vi "Build wash Parameters.vi"(8 "error in (no error)":errorcluster, 10 "Data Controls":T2, 11 "configuration file path":path) -> (0 "error out":errorcluster, 2 "Wash Parameters Array":T1[](array[typedef]) {"Time Target" format="%0.2f"; "Car Position Slider" max=3 scale=0.0..4.0})   [LabVIEW 2015]
doc: "VI used to set parameters for each wash option chosen by the user and build and array output."
uses:
  controls/UI Data.ctl
  controls/Washing Option Parameters.ctl
  <vilib>/Utility/config.llb/Read Key (U32).vi
  <vilib>/Utility/config.llb/Read Key (Double).vi
  <vilib>/Utility/config.llb/NI_LVConfig.lvlib
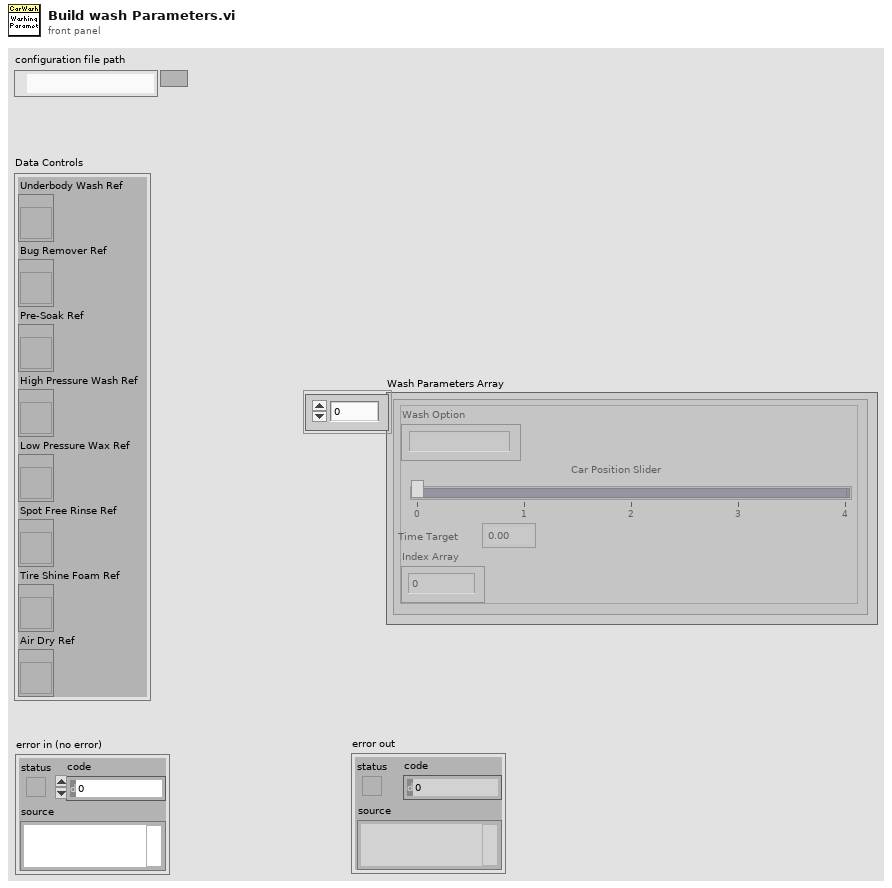
[diagram p1: front panel]
types:
  T1 = typedef "Washing Option Parameters.ctl" = cluster{"Wash Option":string, "Car Position Slider":u8, "Time Target":dbl, "Index Array":i32}
  T2 = typedef "UI Data.ctl" = cluster{"Underbody Wash Ref":refnum<vi>, "Bug Remover Ref":refnum<vi>, "Pre-Soak Ref":refnum<vi>, "High Pressure Wash Ref":refnum<vi>, "Low Pressure Wax Ref":refnum<vi>, "Spot Free Rinse Ref":refnum<vi>, "Tire Shine Foam Ref":refnum<vi>, "Air Dry Ref":refnum<vi>}
  T3 = typedef "NI_LVConfig.lvlib/Config Data RefNum.ctl" = refnum<k1>
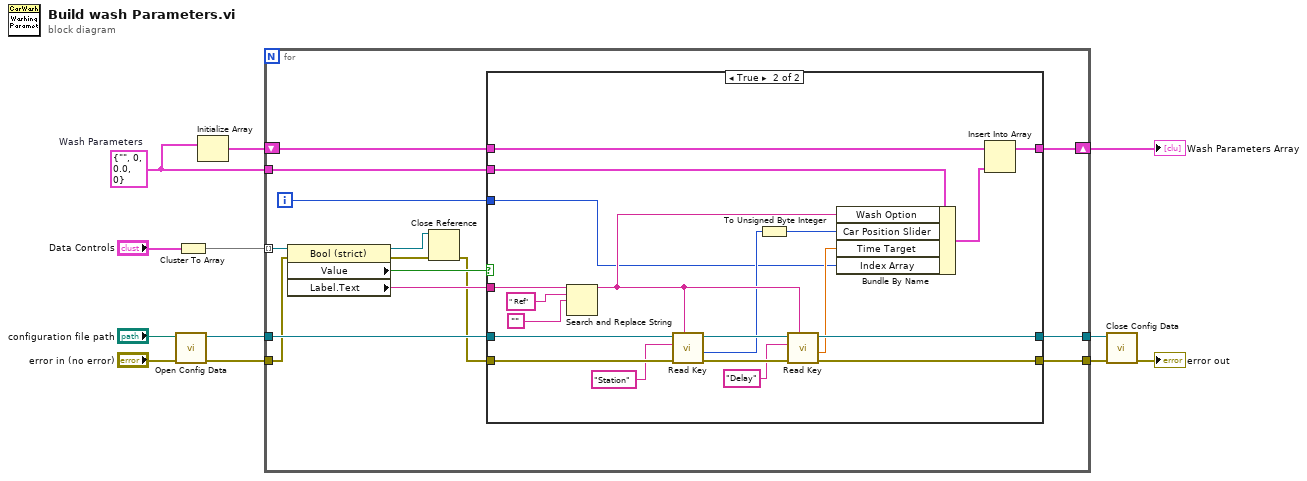
[diagram p0: block diagram]
diagram:
  w6 = T1 {"Wash Option"="", "Car Position Slider"=0, "Time Target"=0.0, "Index Array"=0}  # Wash Parameters
  n1 = call <vilib>:"Open Config Data.vi"("error in (no error)"="error in (no error)", "configuration file path"="configuration file path") -> ("error out"=w10:errorcluster, "refnum"=w11:T3)  [unwired: 7 in, 1 out]
  n2 = Cluster To Array(cluster="Data Controls") -> (array=w1:refnum<vi>[])
  n3 = Initialize Array(w6) -> (w7:T1[])  [unwired: 1 in]
  n4 = for {
    tunnel: w1 -> [w26] mode=indexing
    tunnel: w11 -> [w23]
    tunnel: w10 -> [w14]
    tunnel: [w22] -> w9
    tunnel: [w21] -> w8
    shift-right: [w18] -> w5
    shift-left: w7 -> [w19]
    tunnel: w6 -> [w20]
    i -> [w13]
    n5 = property class="Bool (strict)"(reference=w26, error in=w14) -> (reference out=w15:refnum<vi>, error out=w17:errorcluster, "Value"=w25:bool, "Label.Text"=w24:string)
    n6 = Close Reference(reference=w15, error in (no error)=w17) -> (error out=w16:errorcluster)
    n7 = case shown="True" w25 {
      tunnel: w24 -> [_ w48]
      tunnel: w23 -> [w29 w46]
      tunnel: w16 -> [w28 w44]
      tunnel: [w28 w40] -> w22
      tunnel: [w29 w39] -> w21
      tunnel: w20 -> [_ w38]
      tunnel: w19 -> [w27 w33]
      tunnel: [w27 w31] -> w18
      tunnel: w13 -> [_ w30]
      frame False {
      }
      frame True {
        n8 = Search and Replace String(input string=w48, search string=" Ref" ("substring (\"\")"), replace string="") -> (result string=w37:string)  [unwired: 5 in, 3 out]
        n9 = call-poly <vilib>:"Read Key.vi"("section"=w37, "error in (no error)"=w44, "key"="Station", "refnum"=w46) -> ("error out"=w42:errorcluster, "value"=w35:u32, "refnum out"=w45:T3)  [unwired: 4 in, 1 out]
        n10 = To Unsigned Byte Integer(number=w35) -> (unsigned 8bit integer=w34:u8)
        n11 = call-poly <vilib>:"Read Key.vi"("section"=w37, "error in (no error)"=w42, "key"="Delay", "refnum"=w45) -> ("error out"=w40:errorcluster, "value"=w36:dbl, "refnum out"=w39:T3)  [unwired: 4 in, 1 out]
        n12 = Bundle By Name(cluster=w38, "Wash Option"=w37, "Car Position Slider"=w34, "Time Target"=w36, "Index Array"=w30) -> (w32:T1)
        n13 = Insert Into Array(array=w33, new element=w32) -> (w31:T1[])  [unwired: 1 in]
      }
    }
  }
  "Wash Parameters Array" <- w5
  n14 = call <vilib>:"Close Config Data.vi"("error in (no error)"=w9, "refnum"=w8) -> ("error out"=→"error out":errorcluster)  [unwired: 8 in, 1 out]
